vi "set_heater_spinner.vi"(7 "Remote":bool=TRUE, 8 "Spinner":bool, 9 "Heater":bool) -> ()   [LabVIEW 2011]
uses:
  low_level_proc/globals.vi
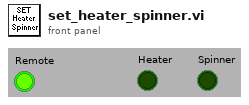
[diagram p1: front panel]
types:
  T1 = typedef "relaySpec.ctl" = cluster{"Card Index":u16, "Relay Index":u16}
  T2 = cluster{"Relay Functions":cluster{"Remote":T1, "Heater on":T1, "Spinner on":T1}}
  T3 = cluster{"Remote":T1, "Heater on":T1, "Spinner on":T1}
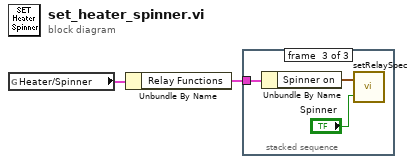
[diagram p0: block diagram]
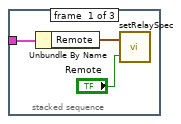
[diagram p2: hidden frame]
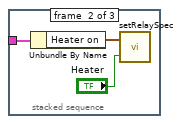
[diagram p3: hidden frame]
diagram:
  n1 = global read "globals.vi" "Heater/Spinner"() -> (w2:T2)
  n2 = Unbundle By Name(w2) -> ("Relay Functions"=w1:T3)
  n3 = stacked-sequence {
    tunnel: w1 -> [w4 w7 w11]
    frame #0 {
      n4 = Unbundle By Name(w4) -> ("Remote"=w3:T1)
      n5 = call "setRelaySpec.vi"("Relay Status"="Remote", "RelaySpec"=w3) -> ()  [unwired: 1 in]
    }
    frame #1 {
      n6 = Unbundle By Name(w7) -> ("Heater on"=w6:T1)
      n7 = call "setRelaySpec.vi"("Relay Status"="Heater", "RelaySpec"=w6) -> ()  [unwired: 1 in]
    }
    frame #2 {
      n8 = Unbundle By Name(w11) -> ("Spinner on"=w10:T1)
      n9 = call "setRelaySpec.vi"("Relay Status"="Spinner", "RelaySpec"=w10) -> ()  [unwired: 1 in]
    }
  }
